vi "Read Datos In.vi"(8 "error in (no error)":errorcluster, 11 "Class 2 in":refnum<class "Class 2.lvclass">) -> (0 "error out":errorcluster, 3 "Class 2 out":refnum<class "Class 2.lvclass">)   [LabVIEW 2019, in "Class 2.lvclass"]
uses:
  Class 2.lvclass
  Class 2.lvclass/Class 2.ctl
  Datos In.vi
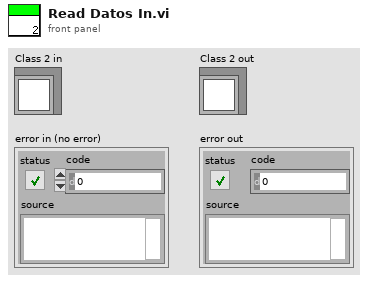
[diagram p1: front panel]
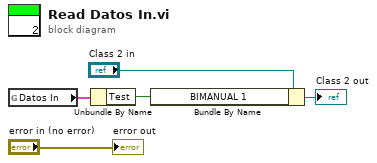
[diagram p0: block diagram]
diagram:
  n1 = global read "Datos In.vi" "Datos In"() -> (w1:cluster{"Test":bool})
  n2 = Unbundle By Name(w1) -> ("Test"=w3:bool)
  n3 = Bundle By Name(cluster="Class 2 in", "BIMANUAL 1"=w3) -> (→"Class 2 out":refnum<class "Class 2.lvclass">)
  "error out" <- "error in (no error)"
